vi "LM Single Exponential and gradient.vi"(3 "output control":T1, 4 "data":variant, 5 "X":dbl[](array[numeric]), 6 "a":dbl[](array[numeric])) -> (0 "error out":errorcluster, 1 "f'(X,a)":dbl[][](array[numeric]), 2 "f(X,a)":dbl[](array[numeric]))   [LabVIEW 2019]
doc: "This template is the starting point for creating a model function to be passed to the Nonlinear Curve Fit.vi."
uses:
  <vilib>/gmath/NumericalOptimization/LM_output select.ctl
  <vilib>/gmath/NI_Gmath.lvlib
panel:
  # "Parameters:\n\nA, t"
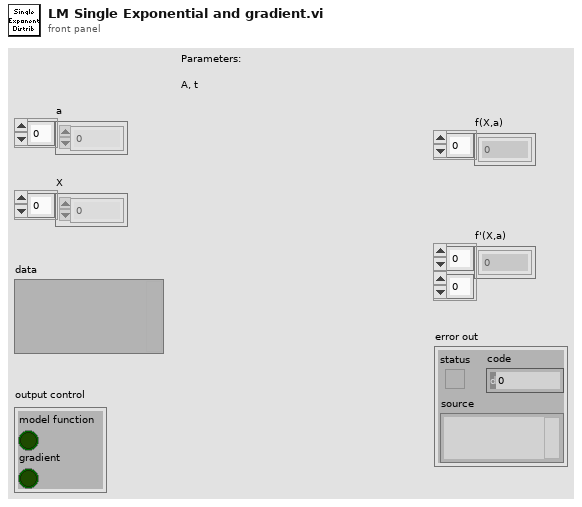
[diagram p1: front panel]
types:
  T1 = typedef "NI_Gmath.lvlib/LM_output select.ctl" = cluster{"model function":bool, "gradient":bool}
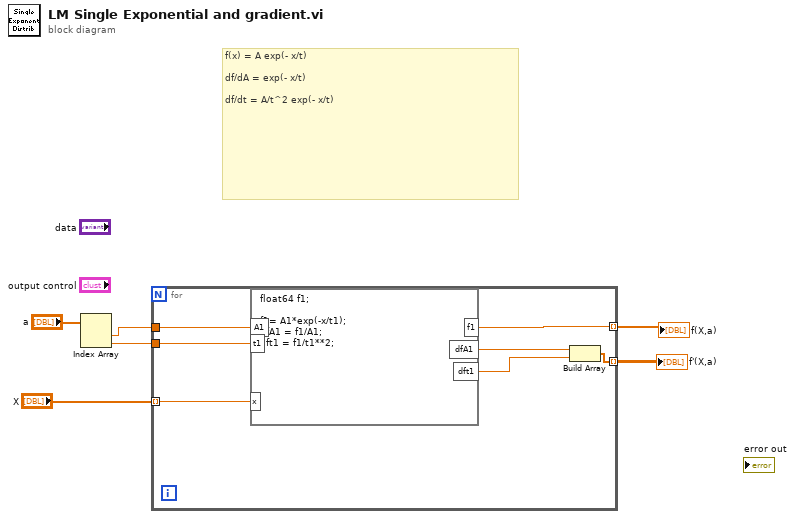
[diagram p0: block diagram]
diagram:
  # "f(x) = A exp(- x/t) \n\ndf/dA = exp(- x/t)     \n\ndf/dt = A/t^2 exp(- x/t)"
  n1 = Index Array(array="a") -> (element #1=w5:dbl, element #2=w4:dbl)  [unwired: 2 in]
  n2 = for {
    tunnel: w5 -> [w13]
    tunnel: w4 -> [w12]
    tunnel: "X" -> [w11] mode=indexing
    tunnel: [w9] -> w2 mode=indexing
    tunnel: [w7] -> w1 mode=indexing
    n3 = formula code="float64 f1;\n\nf1= A1*exp(-x/t1);\ndfA1 = f1/A1;\ndft1 = f1/t1**2;"("A1"=w13, "t1"=w12, "x"=w11) -> ("f1"=w9:dbl, "dfA1"=w10:dbl, "dft1"=w8:dbl)
    n4 = Build Array(w10, w8) -> (w7:dbl[])
  }
  "f(X,a)" <- w2
  "f'(X,a)" <- w1
